vi "Get Class Inheritance from Class Path.vi"(8 "error in (no error)":errorcluster, 11 "lvclass file Path":path) -> (0 "error out":errorcluster, 3 "Class Inheritance [ ]":path[](array[path]))   [LabVIEW 2011, in "VITesterUtilities.lvlib"]
uses:
  Libraries/VITesterUtilities.lvlib
  <vilib>/Utility/lvfile.llb/LVFileType.ctl
  <userlib>/_OpenG.lib/file/file.llb/File Exists - Scalar__ogtk.vi
  <userlib>/_OpenG.lib/file/file.llb/Valid Path - Traditional__ogtk.vi
  <userlib>/_OpenG.lib/array/array.llb/Conditional Auto-Indexing Tunnel (Path)__ogtk.vi
  <userlib>/_OpenG.lib/file/file.llb/Append Path to Root if Relative - Scalar__ogtk.vi
  <vilib>/Utility/lvfile.llb/NI_FileType.lvlib
panel:
  # "Copyright © 2008 James Kring, Inc. All rights reserved.\n\nAuthor: Philippe Guerit [philippe.guerit@jameskring.com]\n             [alternate email: PJM_LabVIEW@yahoo.com]\n\nThis library is provided \"AS IS\" ,WITHOUT WARRANTIES OR \nCONDITIONS OF ANY KIND, either express or implied.\n\nJames Kring, Inc. -- http://www.jameskring.com"
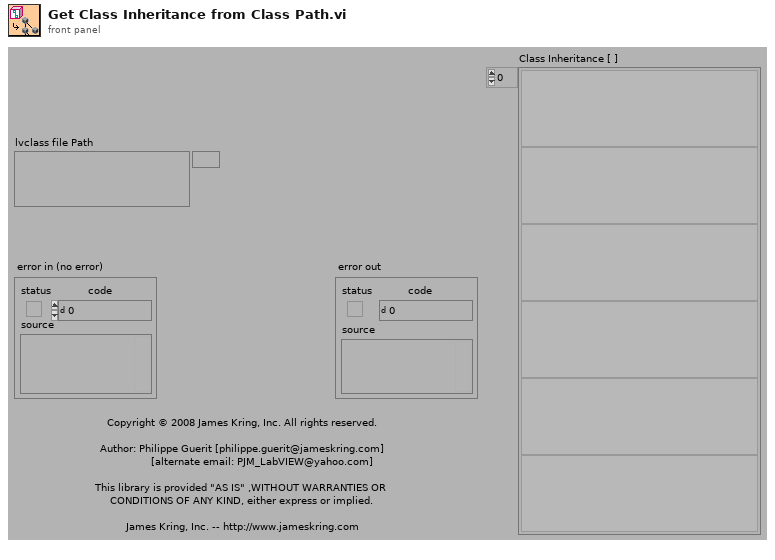
[diagram p1: front panel]
types:
  T1 = typedef "NI_FileType.lvlib/LVFileType.ctl" = enum32{"Invalid file", "Unknown type", "Instrument", "Control", "Polymorphic VI", "Project", "Library", "LVClass", "XControl", "XNode", "Shared library", ".NET assembly", "ActiveX interface", "CIN", "Run-time menu", "Palette menu", "Help file", "LLB", "XNode Edit Dependency", "Class Private Data Control", "Statechart", "MathScript .m file", "Ladder Diagram", "LVLibp"}
  T2 = cluster{"path":path, "delimited name":string, "type":T1, "iState":u32, "iStyle":u16, "wStyle":u16, "buttons":u16, "viflags":u32, "viflags2":u32, "links":u32[]}[]
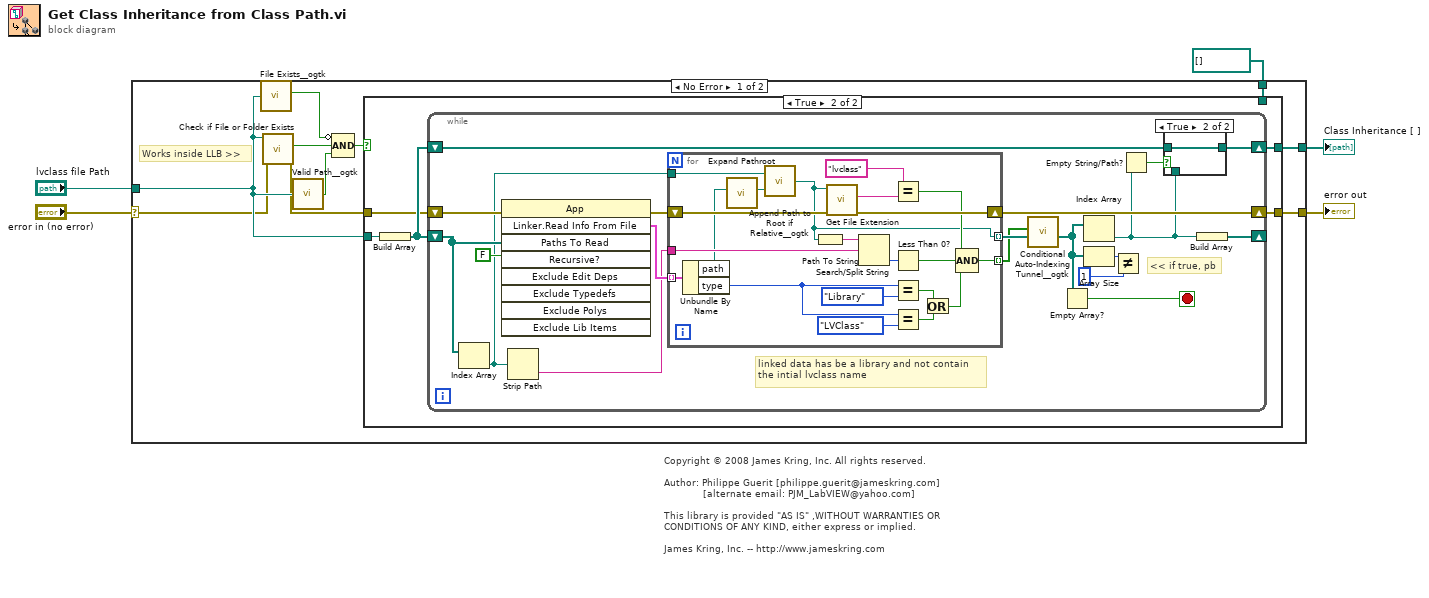
[diagram p0: block diagram]
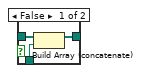
[diagram p3: hidden frame]
diagram:
  # "Copyright © 2008 James Kring, Inc. All rights reserved.\n\nAuthor: Philippe Guerit [philippe.guerit@jameskring.com]\n             [alternate email: PJM_LabVIEW@yahoo.com]\n\nThis library is provided \"AS IS\" ,WITHOUT WARRANTIES OR \nCONDITIONS OF ANY KIND, either express or implied.\n\nJames Kring, Inc. -- http://www.jameskring.com"
  n1 = case shown="No Error" "error in (no error)" {
    selector: "error in (no error)" -> [w7 w68]
    tunnel: [w15 w67] -> w5
    tunnel: "lvclass file Path" -> [w8 _]
    tunnel: [w14 w68] -> w2
    tunnel: path[] [] -> [w10 w67]
    frame No Error {
      # "Works inside LLB >>"
      n2 = call-poly <userlib>:"File Exists__ogtk.vi"("file path"=w8) -> ("is directory"=w13:bool)  [unwired: 6 in, 1 out]
      n3 = call <vilib>:"Check if File or Folder Exists.vi"("error in (no error)"=w7, "path"=w8) -> ("error out"=w6:errorcluster, "file or folder exists?"=w9:bool)  [unwired: 7 in, 1 out]
      n4 = call-poly <userlib>:"Valid Path__ogtk.vi"("path"=w8) -> ("valid"=w12:bool)
      n5 = Compound Arithmetic op=AND(invert w13, w9, w12) -> (w11:bool)
      n6 = case shown="True" w11 {
        tunnel: [w16 w21] -> w15
        tunnel: w6 -> [w17 w20]
        tunnel: [w17 w19] -> w14
        tunnel: w8 -> [_ w18]
        tunnel: w10 -> [w16 _]
        frame False {
        }
        frame True {
          n7 = Build Array(w18) -> (w22:path[])
          n8 = while {
            shift-right: [w29] -> _
            shift-left: w22 -> [w30]
            shift-right: [w31] -> w21
            shift-left: w22 -> [w32]
            shift-right: [w26] -> w19
            shift-left: w20 -> [w28]
            stop <- w33 stop-if-true
            # "<< if true, pb"
            # "linked data has be a library and not contain\nthe intial lvclass name"
            n9 = Index Array(array=w30) -> (element=w23:path)  [unwired: 1 in]
            n10 = invoke class="App" method="Linker.Read Info From File"(error in=w28, "Paths To Read"=w30, "Recursive?"=FALSE) -> (error out=w27:errorcluster, "Linker.Read Info From File"=w40:T2)  [unwired: 6 in, 7 out]
            n11 = Strip Path(path=w23) -> (name=w39:string)  [unwired: 1 out]
            n12 = for {
              tunnel: w40 -> [w66] mode=indexing
              tunnel: w39 -> [w63]
              tunnel: [w51] -> w38 mode=indexing
              tunnel: [w60] -> w37 mode=indexing
              shift-right: [w58] -> w26
              shift-left: w27 -> [w59]
              tunnel: w23 -> [w53]
              n13 = Unbundle By Name(w66) -> ("path"=w52:path, "type"=w49:T1)
              n14 = call "Expand Pathroot.vi"("Path"=w52) -> ("Path out"=w54:path)  [unwired: 10 in]
              n15 = call-poly <userlib>:"Append Path to Root if Relative__ogtk.vi"("Absolute or Relative Path"=w54, "Root Path"=w53) -> ("Absolute or Appended Path"=w51:path)
              n16 = Path To String(path=w51) -> (string=w64:string)
              n17 = call <vilib>:"Get File Extension.vi"("error in (no error)"=w59, "file"=w51) -> ("error out"=w58:errorcluster, "lowercase file extension"=w55:string)  [unwired: 8 out]
              n18 = Search/Split String(string=w64, search string/char (-)=w63) -> (offset of match=w62:i32)  [unwired: 3 out]
              n19 = Equal?(x="lvclass", y=w55) -> (x = y?=w56:bool)
              n20 = Less Than 0?(x=w62) -> (x < 0?=w61:bool)
              n21 = Equal?(x=w49, y=LVFileType."Library") -> (x = y?=w47:bool)
              n22 = Equal?(x=w49, y=LVFileType."LVClass") -> (x = y?=w48:bool)
              n23 = Or(x=w47, y=w48) -> (x .or. y?=w46:bool)
              n24 = Compound Arithmetic op=AND(w56, w61, w46) -> (w60:bool)
            }
            n25 = call-poly <userlib>:"Conditional Auto-Indexing Tunnel__ogtk.vi"("Array in"=w38, "Elements to keep"=w37) -> ("Filtered Array out"=w34:path[])  [unwired: 5 out]
            n26 = Empty Array?(array=w34) -> (empty?=w33:bool)
            n27 = Index Array(array=w34) -> (element=w25:path)  [unwired: 1 in]
            n28 = Array Size(array=w34) -> (size(s)=w36:i32)
            n29 = Not Equal?(x=w36, y=1) -> ()  [unwired: 1 out]
            n30 = Empty String/Path?(string/path=w25) -> (empty?=w24:bool)
            n31 = case shown="True" w24 {
              tunnel: w32 -> [w44 w45]
              tunnel: [w43 w45] -> w31
              tunnel: w25 -> [w42 _]
              frame False {
                n32 = Build Array (concatenate)(w44, w42) -> (w43:path[])
              }
              frame True {
              }
            }
            n33 = Build Array(w25) -> (w29:path[])
          }
        }
      }
    }
    frame Error {
    }
  }
  "Class Inheritance [ ]" <- w5
  "error out" <- w2
